vi "LED.vi"() -> ()   [LabVIEW 2023]
uses:
  <vilib>/Rock Robotics/WPI/Joystick/XBox Buttons Indexer.ctl
  <vilib>/Rock Robotics/WPI/DriverStation/WPI_DriverStationRobotMode2.ctl
  <vilib>/Rock Robotics/WPI/Utilities/WPI_GetSetVariantRefNum.vi
  Framework/Robot Global Data.vi
panel:
  in  "Color 8":u32(colorbox)=16711935
  in  "Color 7":u32(colorbox)=11403496
  in  "Color 6":u32(colorbox)=16860
  in  "Color 5":u32(colorbox)=65535
  in  "Color 4":u32(colorbox)=65280
  in  "Color 3":u32(colorbox)=16776960
  in  "Color 2":u32(colorbox)=16744448
  in  "Color":u32(colorbox)=16711680
  out "output array":u32[](array[numeric])
  out "Current Value":dbl
  out "error out":errorcluster
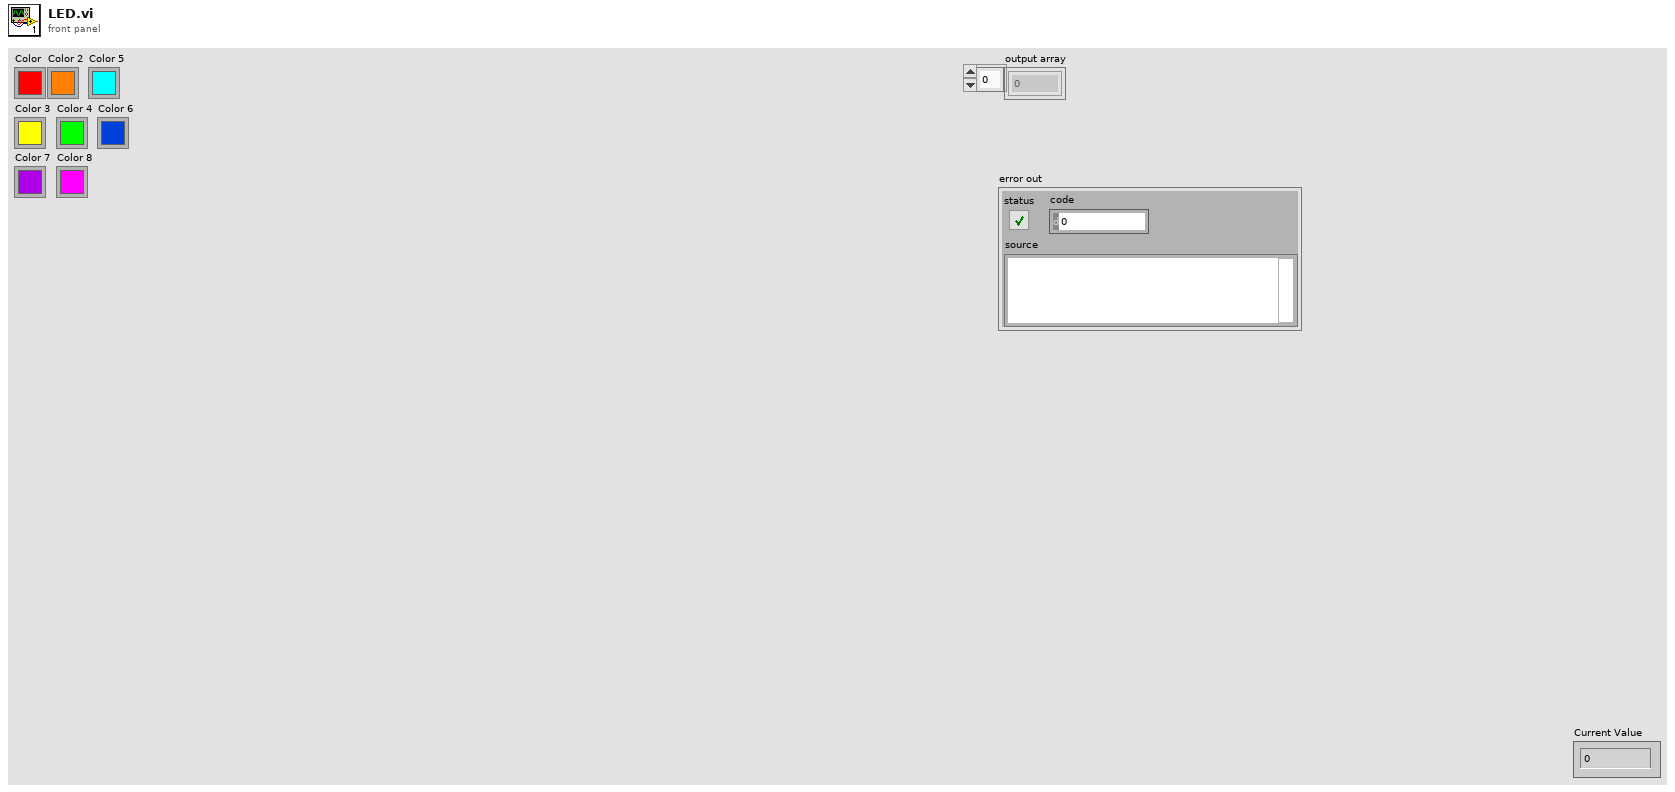
[diagram p1: front panel]
types:
  T1 = typedef "XBox Buttons Indexer.ctl" = enum16{"A", "B", "X", "Y", "Left Bumper", "Right Bumper", "Back", "Start", "Left Joystick", "Right Joystick"}
  T2 = typedef "WPI_DriverStationRobotMode2.ctl" = enum16{"Autonomous Disabled", "Autonomous Enabled", "Teleop Disabled", "Teleop Enabled", "Disconnected", "Finish", "Test Disabled", "Test Enabled", "Emergency Stopped"}
  T3 = typedef "WPI_DriverStationAllianceInfo.ctl" = enum16{"Red", "Blue", "Invalid"}
  T4 = enum16{"Station?", "Transfer", "Node 2", "Node 1", "Node 0"}
  T5 = typedef "WPI_JoystickDevRef.ctl" = cluster{"Device":T6}
  T6 = typedef "WPI_JoystickDeviceEnum.ctl" = enum16{"USB 0", "USB 1", "USB 2", "USB 3", "USB 4", "USB 5"}
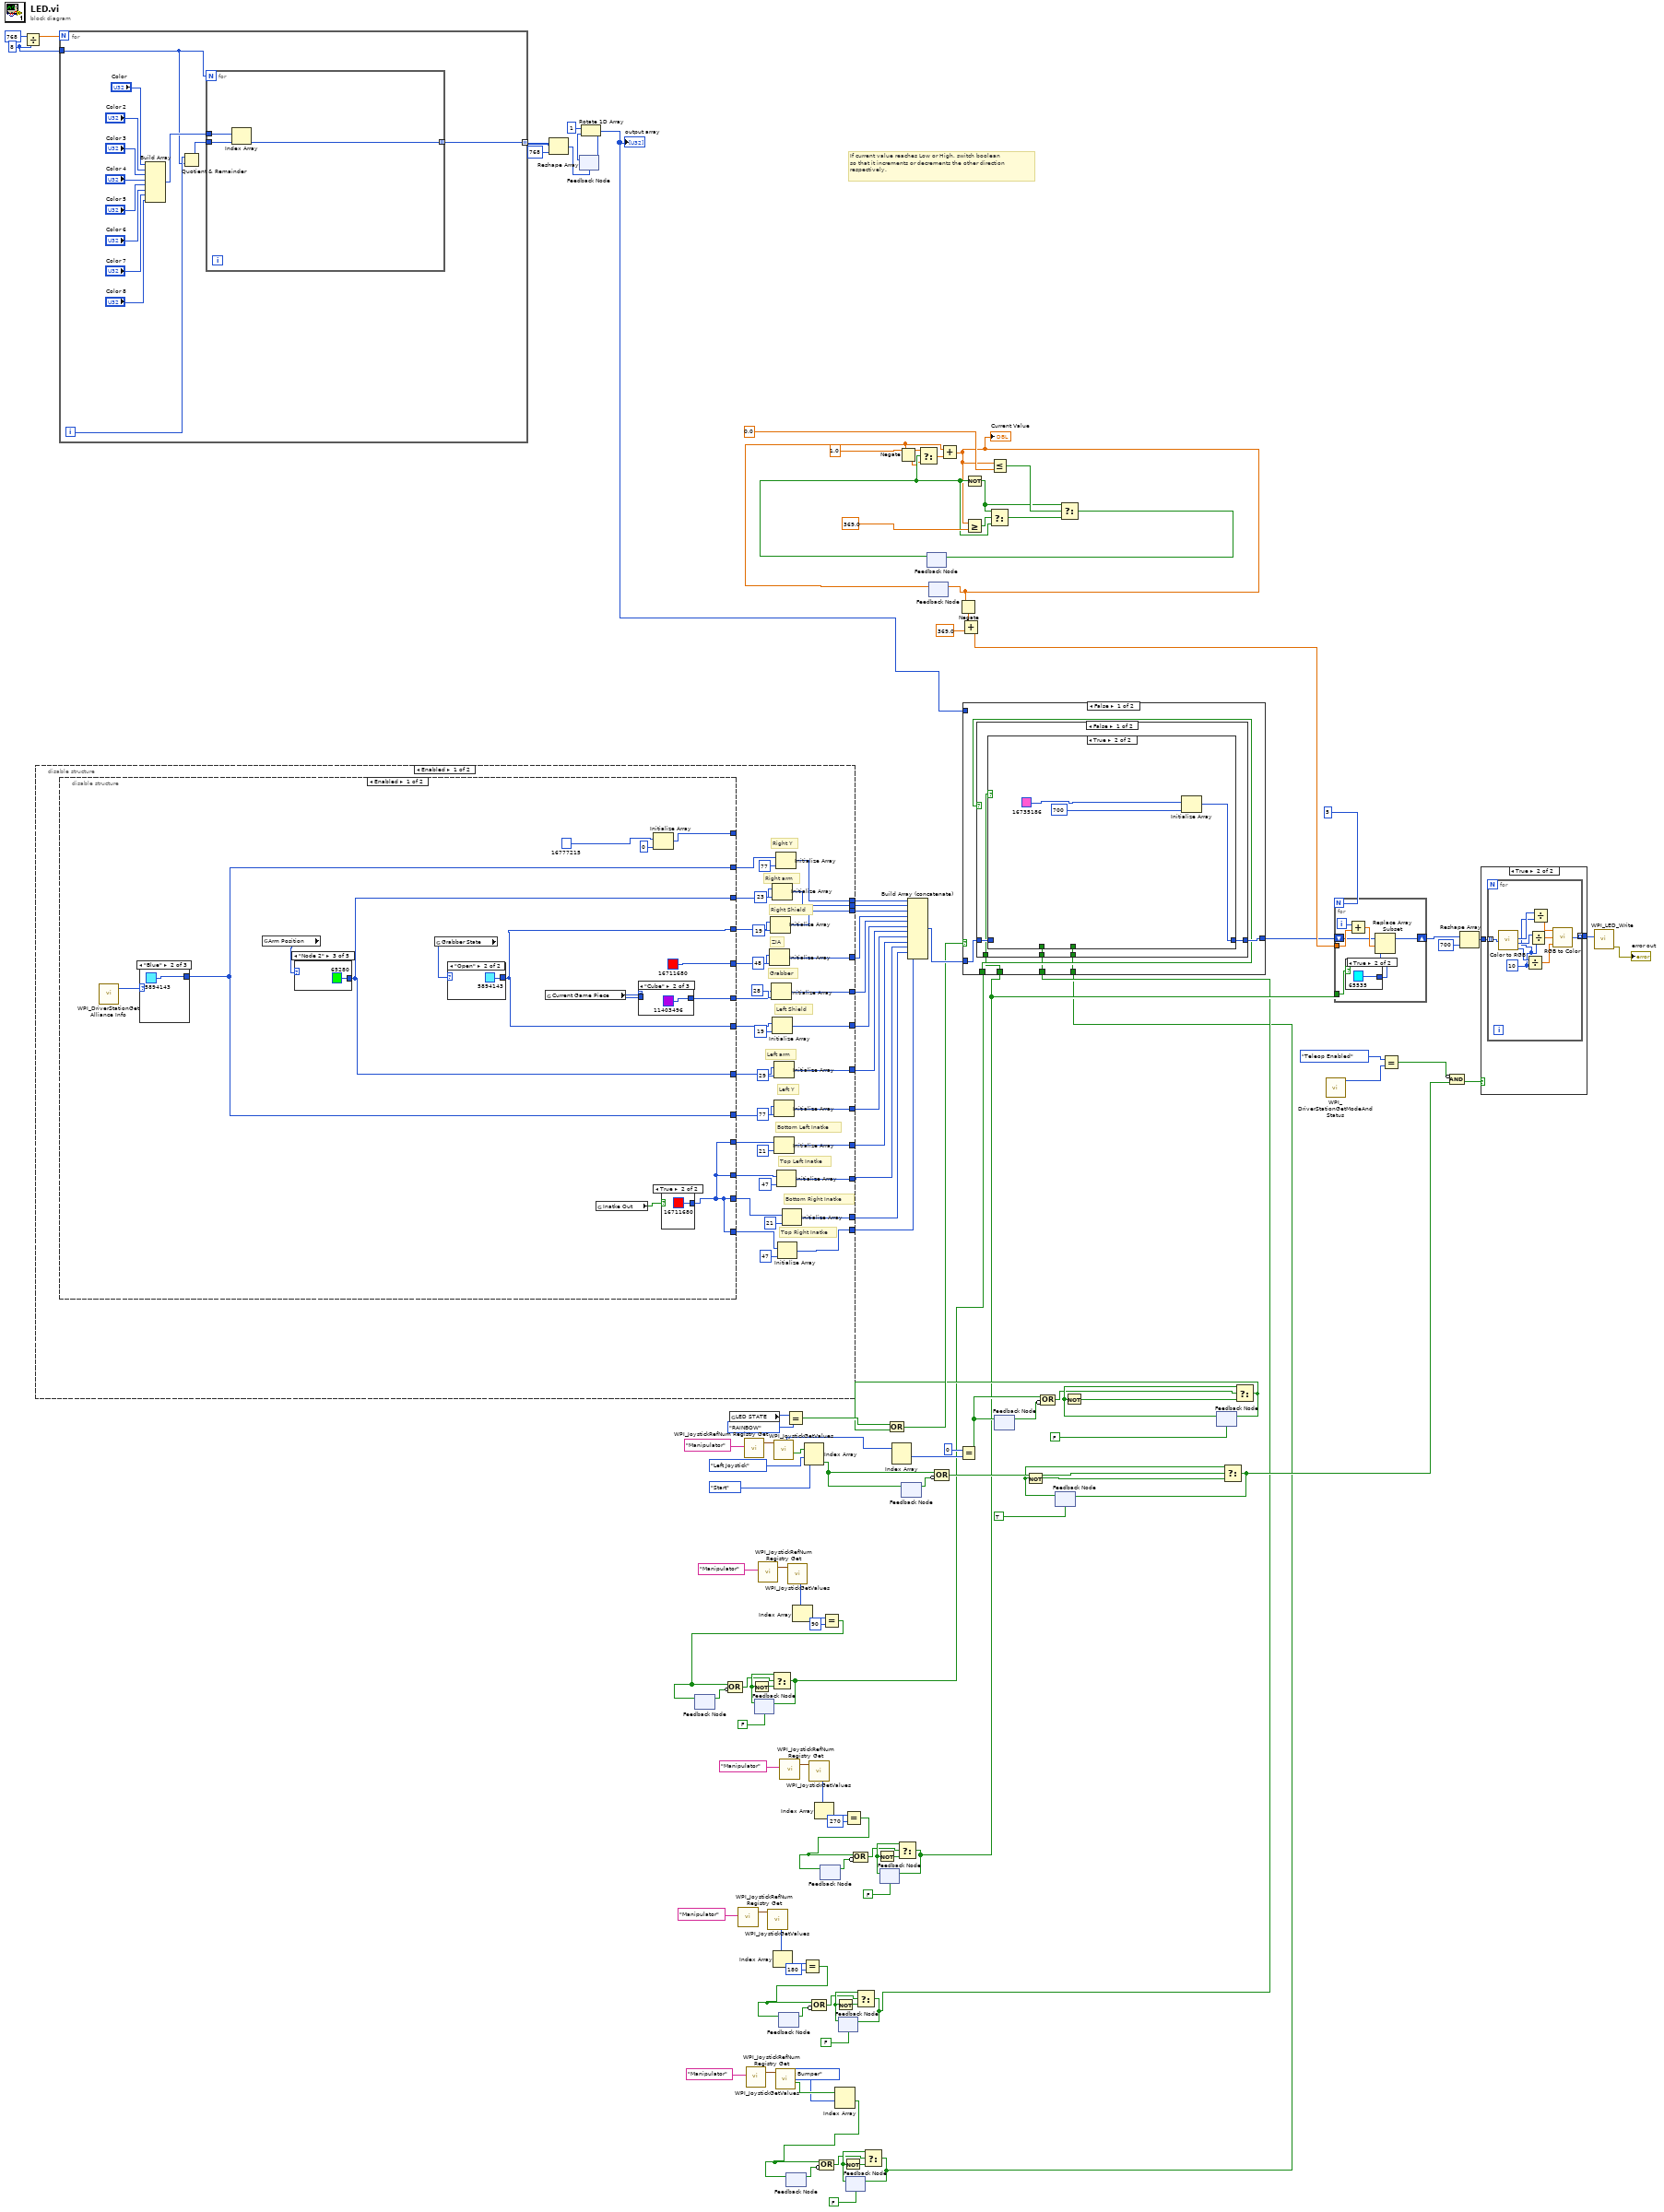
[diagram p0: block diagram]
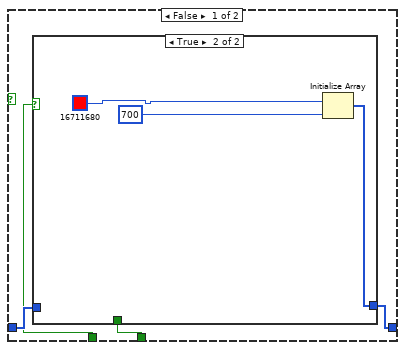
[diagram p3: hidden frame]
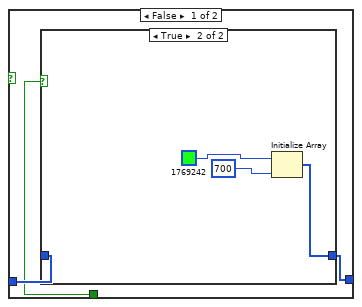
[diagram p4: hidden frame]
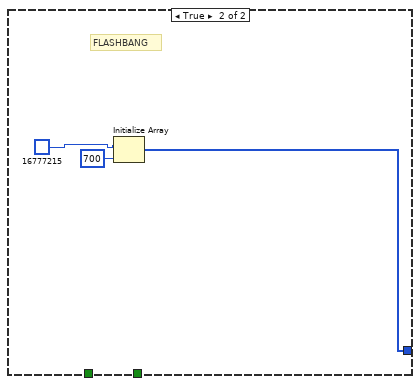
[diagram p6: hidden frame]
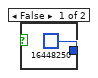
[diagram p8: hidden frame]
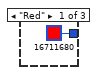
[diagram p9: hidden frame]
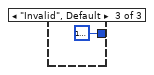
[diagram p10: hidden frame]
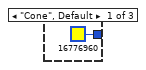
[diagram p11: hidden frame]
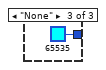
[diagram p12: hidden frame]
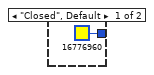
[diagram p13: hidden frame]
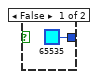
[diagram p14: hidden frame]
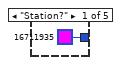
[diagram p15: hidden frame]
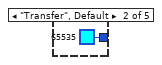
[diagram p16: hidden frame]
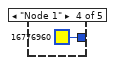
[diagram p17: hidden frame]
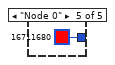
[diagram p18: hidden frame]
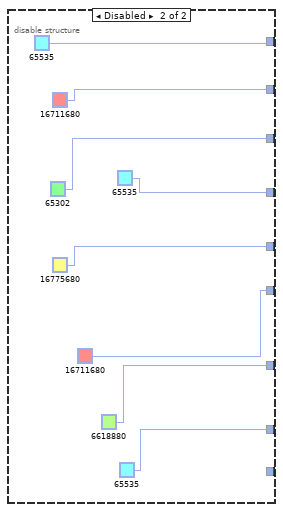
[diagram p19: hidden frame]
diagram:
  w99 = 8 ("y")
  # "If current value reaches Low or High, switch boolean\nso that it increments or decrements the other direction\nrespectively."
  n1 = Divide(x=768, y=w99) -> (x/y=w105:dbl)
  n2 = disable-structure shown="Enabled" {
    disable-tunnel: [w158 _] -> w121
    disable-tunnel: [w157 _] -> w120
    disable-tunnel: [w156 _] -> w83
    disable-tunnel: [w155 _] -> w119
    disable-tunnel: [w145 _] -> w80
    disable-tunnel: [w143 _] -> w4
    disable-tunnel: [w139 _] -> w2
    disable-tunnel: [w131 _] -> w82
    disable-tunnel: [w130 _] -> w84
    disable-tunnel: [w129 _] -> w81
    disable-tunnel: [w127 _] -> w3
    disable-tunnel: [w123 _] -> w1
    frame Enabled {
      # "Top Left Inatke"
      # "Top Right Inatke"
      # "Bottom Right Inatke"
      # "Bottom Left Inatke"
      # "Left Y"
      # "Left arm"
      # "Left Shield"
      # "Grabber"
      # "ZIA"
      # "Right Shield"
      # "Right arm"
      # "Right Y"
      n3 = disable-structure shown="Enabled" {
        disable-tunnel: [w168 u32 16711680 ("Color")] -> w149
        disable-tunnel: [w172 u32 16775680 ("Color")] -> w147
        disable-tunnel: [w159 _] -> w141
        disable-tunnel: [w169 u32 6618880 ("Color")] -> w137
        disable-tunnel: [u32 16711680 ("Color") u32 65535 ("Color")] -> w136
        disable-tunnel: [w170 u32 65535 ("Color")] -> w135
        disable-tunnel: [w170 u32 65535 ("Color")] -> w134
        disable-tunnel: [w169 u32 16711680 ("Color")] -> w133
        disable-tunnel: [w168 u32 65302 ("Color")] -> w132
        disable-tunnel: [w167 _] -> _
        disable-tunnel: [w159 _] -> w126
        disable-tunnel: [w159 _] -> w125
        disable-tunnel: [w159 _] -> w124
        frame Enabled {
          n4 = call <vilib>:"WPI_DriverStationGet Alliance Info.vi"() -> ("Alliance"=w162:T3)  [unwired: 6 in, 5 out]
          n5 = case shown="\"Blue\"" w162 {
            tunnel: [u32 16711680 ("Color") u32 5894143 ("Color") u32 16777225 ("Color")] -> w170
            frame "Red" {
            }
            frame "Blue" {
            }
            frame "Invalid", Default {
            }
          }
          n6 = global read "Robot Global Data.vi" "Arm Position"() -> (w166:T4)
          n7 = case shown="\"Node 2\"" w166 {
            tunnel: [u32 16711935 ("Color") u32 65535 ("Color") u32 65280 ("Color") u32 16776960 ("Color") u32 16711680 ("Color")] -> w169
            frame "Station?" {
            }
            frame "Transfer", Default {
            }
            frame "Node 2" {
            }
            frame "Node 1" {
            }
            frame "Node 0" {
            }
          }
          n8 = global read "Robot Global Data.vi" "Grabber State"() -> (w164:enum16{"Closed", "Open"})
          n9 = case shown="\"Open\"" w164 {
            tunnel: [u32 16776960 ("Color") u32 5894143 ("Color")] -> w168
            frame "Closed", Default {
            }
            frame "Open" {
            }
          }
          n10 = global read "Robot Global Data.vi" "Current Game Piece"() -> (w163:enum16{"Cone", "Cube", "None"})
          n11 = global read "Robot Global Data.vi" "Inatke Out"() -> (w165:bool)
          n12 = case shown="\"Cube\"" w163 {
            tunnel: [u32 16776960 ("Color") u32 11403496 ("Color") u32 65535 ("Color")] -> w172
            tunnel: w163 -> [_ _ _]
            frame "Cone", Default {
            }
            frame "Cube" {
            }
            frame "None" {
            }
          }
          n13 = Initialize Array(u32 16777215 ("Color"), 0 ("dimension size")) -> (w167:u32[])
          n14 = case shown="True" w165 {
            tunnel: [u32 65535 ("Color") u32 16711680 ("Color")] -> w159
            frame False {
            }
            frame True {
            }
          }
        }
        frame Disabled {
        }
      }
      n15 = Initialize Array(w136, 48 ("dimension size")) -> (w130:u32[])
      n16 = Initialize Array(w132, 19 ("dimension size")) -> (w155:u32[])
      n17 = Initialize Array(w147, 28 ("dimension size")) -> (w156:u32[])
      n18 = Initialize Array(w133, 23 ("dimension size")) -> (w157:u32[])
      n19 = Initialize Array(w149, 19 ("dimension size")) -> (w129:u32[])
      n20 = Initialize Array(w137, 29 ("dimension size")) -> (w145:u32[])
      n21 = Initialize Array(w134, 77 ("dimension size")) -> (w131:u32[])
      n22 = Initialize Array(w126, 21 ("dimension size")) -> (w143:u32[])
      n23 = Initialize Array(w135, 77 ("dimension size")) -> (w158:u32[])
      n24 = Initialize Array(w125, 47 ("dimension size")) -> (w127:u32[])
      n25 = Initialize Array(w124, 47 ("dimension size")) -> (w123:u32[])
      n26 = Initialize Array(w141, 21 ("dimension size")) -> (w139:u32[])
    }
    frame Disabled {
    }
  }
  n27 = for {
    N: w105 -> [_]
    tunnel: [w198] -> w104 mode=indexing
    tunnel: w99 -> [w196]
    i -> [w197]
    n28 = Build Array("Color", "Color 2", "Color 3", "Color 4", "Color 5", "Color 6", "Color 7", "Color 8") -> (w200:u32[])
    n29 = Quotient & Remainder(x=w197, y=w196) -> (x-y*floor(x/y)=w199:i32)  [unwired: 1 out]
    n30 = for {
      N: w196 -> [_]
      tunnel: w200 -> [w211]
      tunnel: w199 -> [w210]
      tunnel: [w209] -> w198 mode=indexing
      n31 = Index Array(array=w211, index=w210) -> (element=w209:u32)
    }
  }
  n32 = Reshape Array(w104, 768 ("dimension size")) -> (w101:u32[])
  n33 = feedback #1(w101) -> (w102:u32[])
  n34 = Rotate 1D Array(1:w102, 2:1 ("n")) -> (0:w89:u32[])
  "output array" <- w89
  n35 = feedback-in #1(w89) -> ()
  n36 = feedback #2() -> (w43:bool)  [unwired: 1 in]
  n37 = global read "Robot Global Data.vi" "LED STATE"() -> (w79:enum16{"NORMAL", "RAINBOW"})
  n38 = call <vilib>:"WPI_JoystickRefNum Registry Get.vi"("refnum name"="Manipulator") -> ("JoystickDevRef"=w26:T5)  [unwired: 1 in, 9 out]
  n39 = call <vilib>:"WPI_JoystickRefNum Registry Get.vi"("refnum name"="Manipulator") -> ("JoystickDevRef"=w92:T5)  [unwired: 1 in, 9 out]
  n40 = call <vilib>:"WPI_JoystickRefNum Registry Get.vi"("refnum name"="Manipulator") -> ("JoystickDevRef"=w10:T5)  [unwired: 1 in, 9 out]
  n41 = feedback #3(FALSE) -> (w44:bool)
  n42 = Not(x=w44) -> (.not. x?=w45:bool)
  n43 = call <vilib>:"WPI_JoystickRefNum Registry Get.vi"("refnum name"="Manipulator") -> ("JoystickDevRef"=w50:T5)  [unwired: 1 in, 9 out]
  n44 = call <vilib>:"WPI_JoystickGetValues.vi"("JoystickDevRef"=w26) -> ("POVs"=w25:i16[])  [unwired: 6 in, 4 out]
  n45 = Index Array(array=w25) -> (element=w24:i16)  [unwired: 1 in]
  n46 = call <vilib>:"WPI_JoystickGetValues.vi"("JoystickDevRef"=w92) -> ("Buttons"=w91:bool[], "POVs"=w61:i16[])  [unwired: 6 in, 3 out]
  n47 = call <vilib>:"WPI_JoystickGetValues.vi"("JoystickDevRef"=w10) -> ("Buttons"=w7:bool[])  [unwired: 6 in, 4 out]
  n48 = feedback #4() -> (w19:bool)  [unwired: 1 in]
  n49 = call <vilib>:"WPI_JoystickRefNum Registry Get.vi"("refnum name"="Manipulator") -> ("JoystickDevRef"=w38:T5)  [unwired: 1 in, 9 out]
  n50 = Equal?(x=w79, y=enum16{"NORMAL", "RAINBOW"}."RAINBOW") -> (x = y?=w76:bool)
  n51 = feedback #5() -> (w12:bool)  [unwired: 1 in]
  n52 = call <vilib>:"WPI_JoystickGetValues.vi"("JoystickDevRef"=w50) -> ("POVs"=w49:i16[])  [unwired: 6 in, 4 out]
  n53 = Index Array(array=w49) -> (element=w48:i16)  [unwired: 1 in]
  n54 = Equal?(x=w24, y=i16 180) -> (x = y?=w17:bool)
  n55 = feedback-in #4(w17) -> ()
  n56 = Index Array(array=w91, index #1=XBox_Buttons_Indexer."Left Joystick" ("XBox Buttons"), index #2=XBox_Buttons_Indexer."Start" ("XBox Buttons")) -> (element #2=w71:bool)  [unwired: 1 out]
  n57 = call <vilib>:"WPI_JoystickGetValues.vi"("JoystickDevRef"=w38) -> ("POVs"=w37:i16[])  [unwired: 6 in, 4 out]
  n58 = Compound Arithmetic op=OR(w17, invert w19) -> (w18:bool)
  n59 = Index Array(array=w37) -> (element=w36:i16)  [unwired: 1 in]
  n60 = feedback #6() -> (w31:bool)  [unwired: 1 in]
  n61 = Equal?(x=w48, y=i16 90) -> (x = y?=w41:bool)
  n62 = feedback-in #2(w41) -> ()
  n63 = Compound Arithmetic op=OR(w41, invert w43) -> (w42:bool)
  n64 = Select(t=w44, s=w42, f=w45) -> (s? t:f=w40:bool)
  n65 = feedback-in #3(w40) -> ()
  n66 = Index Array(array=w7, index #1=XBox_Buttons_Indexer."Left Bumper" ("XBox Buttons")) -> (element #1=w5:bool)  [unwired: 1 in, 1 out]
  n67 = feedback-in #5(w5) -> ()
  n68 = Compound Arithmetic op=OR(w5, invert w12) -> (w11:bool)
  n69 = feedback #7(FALSE) -> (w20:bool)
  n70 = Not(x=w20) -> (.not. x?=w21:bool)
  n71 = Equal?(x=w36, y=i16 270) -> (x = y?=w29:bool)
  n72 = feedback-in #6(w29) -> ()
  n73 = feedback #8(FALSE) -> (w13:bool)
  n74 = Not(x=w13) -> (.not. x?=w14:bool)
  n75 = Compound Arithmetic op=OR(w29, invert w31) -> (w30:bool)
  n76 = Select(t=w20, s=w18, f=w21) -> (s? t:f=w16:bool)
  n77 = feedback-in #7(w16) -> ()
  n78 = Select(t=w13, s=w11, f=w14) -> (s? t:f=w8:bool)
  n79 = feedback-in #8(w8) -> ()
  n80 = feedback #9(FALSE) -> (w32:bool)
  n81 = Not(x=w32) -> (.not. x?=w33:bool)
  n82 = Index Array(array=w61) -> (element #1=w60:i16)  [unwired: 2 in, 1 out]
  n83 = Select(t=w32, s=w30, f=w33) -> (s? t:f=w28:bool)
  n84 = feedback-in #9(w28) -> ()
  n85 = feedback-in #10(w71) -> ()
  n86 = feedback #10() -> (w72:bool)  [unwired: 1 in]
  n87 = Build Array (concatenate)(w121, w120, w119, w84, w83, w81, w80, w82, w4, w3, w2, w1) -> (w87:u32[])
  n88 = feedback #11() -> (w109:bool)  [unwired: 1 in]
  n89 = feedback #12() -> (w108:dbl)  [unwired: 1 in]
  n90 = Negate(x=w108) -> (-x=w107:dbl)
  n91 = Select(t=1.0 ("Increment"), s=w109, f=w107) -> (s? t:f=w116:dbl)
  n92 = Compound Arithmetic op=OR(w71, invert w72) -> (w70:bool)
  n93 = Add(x=w108, y=w116) -> (x+y=w97:dbl)
  "Current Value" <- w97
  n94 = feedback-in #12(w97) -> ()
  n95 = Negate(x=w97) -> (-x=w96:dbl)
  n96 = Equal?(x=i16 0, y=w60) -> (x = y?=w53:bool)
  n97 = Add(x=w96, y=369.0) -> (x+y=w95:dbl)
  n98 = Not(x=w109) -> (.not. x?=w111:bool)
  n99 = Greater Or Equal?(x=w97, y=369.0 ("High")) -> (x >= y?=w115:bool)
  n100 = Less Or Equal?(x=w97, y=0.0 ("Low")) -> (x <= y?=w112:bool)
  n101 = Select(t=w111, s=w115, f=w109) -> (s? t:f=w114:bool)
  n102 = feedback #13() -> (w54:bool)  [unwired: 1 in]
  n103 = feedback-in #13(w53) -> ()
  n104 = Compound Arithmetic op=OR(w53, invert w54) -> (w52:bool)
  n105 = feedback #14(TRUE) -> (w62:bool)
  n106 = Not(x=w62) -> (.not. x?=w63:bool)
  n107 = Select(t=w111, s=w112, f=w114) -> (s? t:f=w110:bool)
  n108 = feedback-in #11(w110) -> ()
  n109 = feedback #15(FALSE) -> (w56:bool)
  n110 = Not(x=w56) -> (.not. x?=w57:bool)
  n111 = Select(t=w62, s=w70, f=w63) -> (s? t:f=w68:bool)
  n112 = feedback-in #14(w68) -> ()
  n113 = Select(t=w56, s=w52, f=w57) -> (s? t:f=w55:bool)
  n114 = Or(x=w76, y=w55) -> (x .or. y?=w77:bool)
  n115 = case shown="False" w77 {
    tunnel: w89 -> [_ w243]
    tunnel: [w217 w243] -> w88
    tunnel: w87 -> [w216 _]
    tunnel: w40 -> [w215 _]
    tunnel: w28 -> [w214 _]
    tunnel: w16 -> [w213 _]
    tunnel: w8 -> [w212 _]
    frame False {
      n116 = case shown="False" w215 {
        tunnel: [w222 w240] -> w217
        tunnel: w216 -> [w221 _]
        tunnel: w214 -> [w220 _]
        tunnel: w213 -> [w219 _]
        tunnel: w212 -> [w218 _]
        frame False {
          n117 = case shown="True" w220 {
            tunnel: [w226 w237] -> w222
            tunnel: w221 -> [w225 _]
            tunnel: w219 -> [w224 _]
            tunnel: w218 -> [w223 _]
            frame False {
              n118 = case shown="True" w224 {
                tunnel: [w228 w234] -> w226
                tunnel: w225 -> [w229 _]
                tunnel: w223 -> [w227 _]
                frame False {
                  n119 = case shown="True" w227 {
                    tunnel: w229 -> [w230 _]
                    tunnel: [w230 w231] -> w228
                    frame False {
                      # "NORMAL"
                    }
                    frame True {
                      n120 = Initialize Array(u32 1769242 ("Color"), 700 ("dimension size")) -> (w231:u32[])
                    }
                  }
                }
                frame True {
                  n121 = Initialize Array(u32 16711680 ("Color"), 700 ("dimension size")) -> (w234:u32[])
                }
              }
            }
            frame True {
              n122 = Initialize Array(u32 16735186 ("Color"), 700 ("dimension size")) -> (w237:u32[])
            }
          }
        }
        frame True {
          # "FLASHBANG"
          n123 = Initialize Array(u32 16777215 ("Color"), 700 ("dimension size")) -> (w240:u32[])
        }
      }
    }
    frame True {
      # "RAINBOW"
    }
  }
  n124 = feedback-in #15(w55) -> ()
  n125 = call <vilib>:"WPI_DriverStationGetModeAndStatus.vi"() -> ("Robot Mode"=w65:T2)  [unwired: 10 in, 1 out]
  n126 = for {
    N: 5 -> [_]
    tunnel: w95 -> [w249]
    shift-right: [w245] -> w86
    shift-left: w88 -> [w246]
    tunnel: w28 -> [w244]
    i -> [w248]
    n127 = case shown="True" w244 {
      tunnel: [u32 16448250 ("Color") u32 65535 ("Color")] -> w250
      frame False {
      }
      frame True {
      }
    }
    n128 = Add(x=w248, y=w249) -> (x+y=w247:dbl)
    n129 = Replace Array Subset(array=w246, new element=w250, index=w247) -> (w245:u32[])
  }
  n130 = Equal?(x=WPI_DriverStationRobotMode2."Teleop Enabled" ("Robot Mode"), y=w65) -> (x = y?=w64:bool)
  n131 = Compound Arithmetic op=AND(invert w64, w68) -> (w67:bool)
  n132 = Reshape Array(w86, 700 ("dimension size")) -> (w74:u32[])
  n133 = case shown="True" w67 {
    tunnel: [w253 w255] -> w75
    tunnel: w74 -> [w253 w254]
    frame False {
    }
    frame True {
      n134 = for {
        tunnel: [w263] -> w255 mode=indexing
        tunnel: w254 -> [w264] mode=indexing
        w256 = u8 10 ("y")
        n135 = call <vilib>:"Color to RGB.vi"("Color"=w264) -> ("R"=w259:u8, "G"=w257:u8, "B"=w258:u8)  [unwired: 1 out]
        n136 = Divide(x=w258, y=w256) -> (x/y=w262:dbl)
        n137 = Divide(x=w257, y=w256) -> (x/y=w261:dbl)
        n138 = Divide(x=w259, y=w256) -> (x/y=w260:dbl)
        n139 = call <vilib>:"RGB to Color.vi"("B"=w262, "G"=w261, "R"=w260) -> ("Color"=w263:u32)
      }
    }
  }
  n140 = call <vilib>:"WPI_LED_Write.vi"("Color Array"=w75) -> ("error out"=→"error out":errorcluster)  [unwired: 10 in]
